vi "release_hw.vi"(8 "error in (no error)":errorcluster, 11 "glaz in":refnum<class "glaz.lvclass">) -> (0 "error out":errorcluster, 3 "glaz out":refnum<class "glaz.lvclass">)   [LabVIEW 2019, in "glaz.lvlib" / "glaz.lvclass"]
uses:
  glaz.lvclass
panel:
  out "return type 2":i32
  out "return type":i32
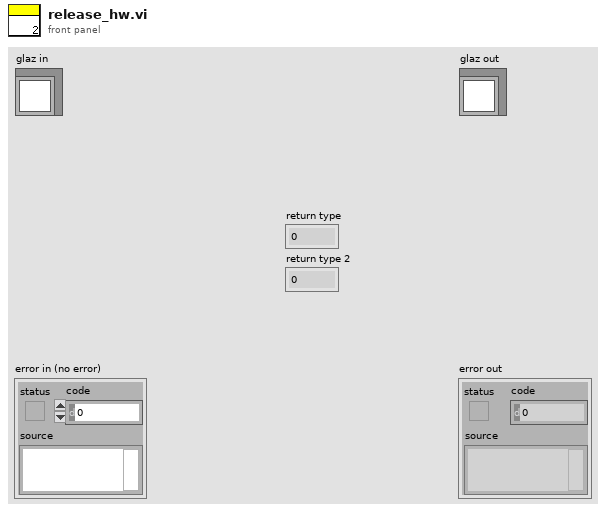
[diagram p1: front panel]
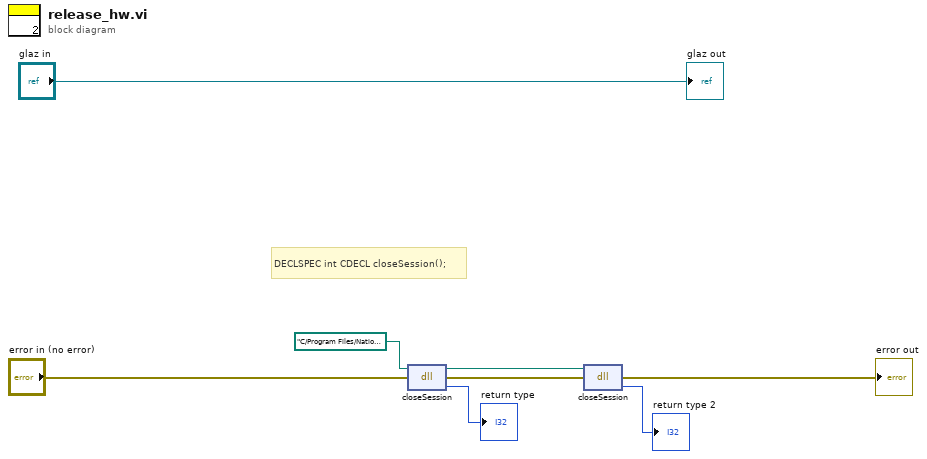
[diagram p0: block diagram]
diagram:
  # "DECLSPEC int CDECL closeSession();"
  n1 = dll-call lib="C:/Program Files/National Instruments/LabVIEW 2019/user.lib/GlazLabView/GlazLib.*" fn="closeSession"(path in=path "C:/Program Files/National Instruments/LabVIEW 2019/user.lib/GlazLabView/GlazLib.*", error in="error in (no error)") -> (path out=w5:path, error out=w4:errorcluster, "return type"=→"return type":i32)  [unwired: 1 in]
  n2 = dll-call lib="C:/Program Files/National Instruments/LabVIEW 2019/user.lib/GlazLabView/GlazLib.*" fn="closeSession"(path in=w5, error in=w4) -> (error out=→"error out":errorcluster, "return type"=→"return type 2":i32)  [unwired: 1 in, 1 out]
  "glaz out" <- "glaz in"
